vi "GetAppOutput.vi"(8 "error in (no error)":errorcluster, 11 "RingdownPlugin in":refnum<class "RingdownPlugin.lvclass">) -> (0 "error out":errorcluster, 3 "RingdownPlugin out":refnum<class "RingdownPlugin.lvclass">)   [LabVIEW 2014, in "AppPlugins.lvlib" / "RingdownPlugin.lvclass"]
uses:
  RingdownPlugin.lvclass
  TypeDef/RingdownOutput.ctl
  RingdownPlugin.lvclass/RingdownPlugin.ctl
  Accessors/Read RingdownConfig.vi
panel:
  out "Warning":i32
  out "Output Parameters":T1
  out "Time of process":dbl
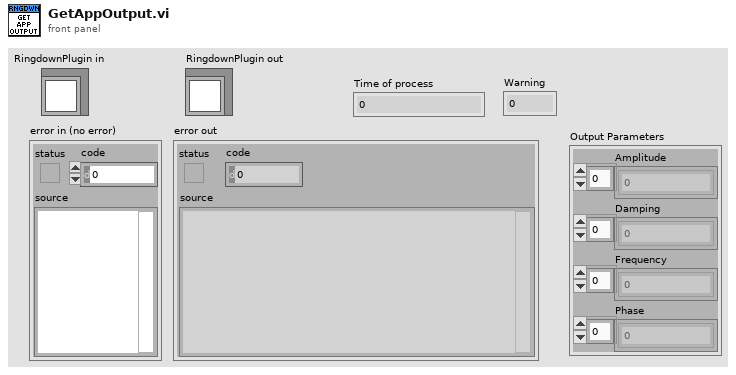
[diagram p1: front panel]
types:
  T1 = cluster{"Amplitude":dbl[], "Damping":dbl[], "Frequency":dbl[], "Phase":dbl[]}
  T2 = typedef "AppPlugins.lvlib/RingdownPlugin.lvclass/RingdownOutput.ctl" = cluster{"FramesPerSecond":dbl, "PronyEstimate":dbl[], "RingdownParameters":cluster{"Amplitude":dbl[], "Damping":dbl[], "Frequency":dbl[], "Phase":dbl[]}, "ReportingTime":dbl, "DataSize":u32, "InputSignal":dbl[]}
  T3 = typedef "AppPlugins.lvlib/RingdownPlugin.lvclass/RingdownConfig.ctl" = cluster{"Config":cluster{"Addmod":i32, "Scalmod":i32, "Lpocon":i32, "Pircon":i32, "Dmodes":i32, "Lpmcon":u16, "Lpacon":u16, "Fbcon":u16, "Ordcon":i32, "Trimre":dbl, "Ftrimh":dbl, "Ftriml":dbl}, "Window":cluster{"StOffset":i32, "EndOffset":i32, "Length":i32}, "V index":i32, "I index":i32, "PosSeq":bool}
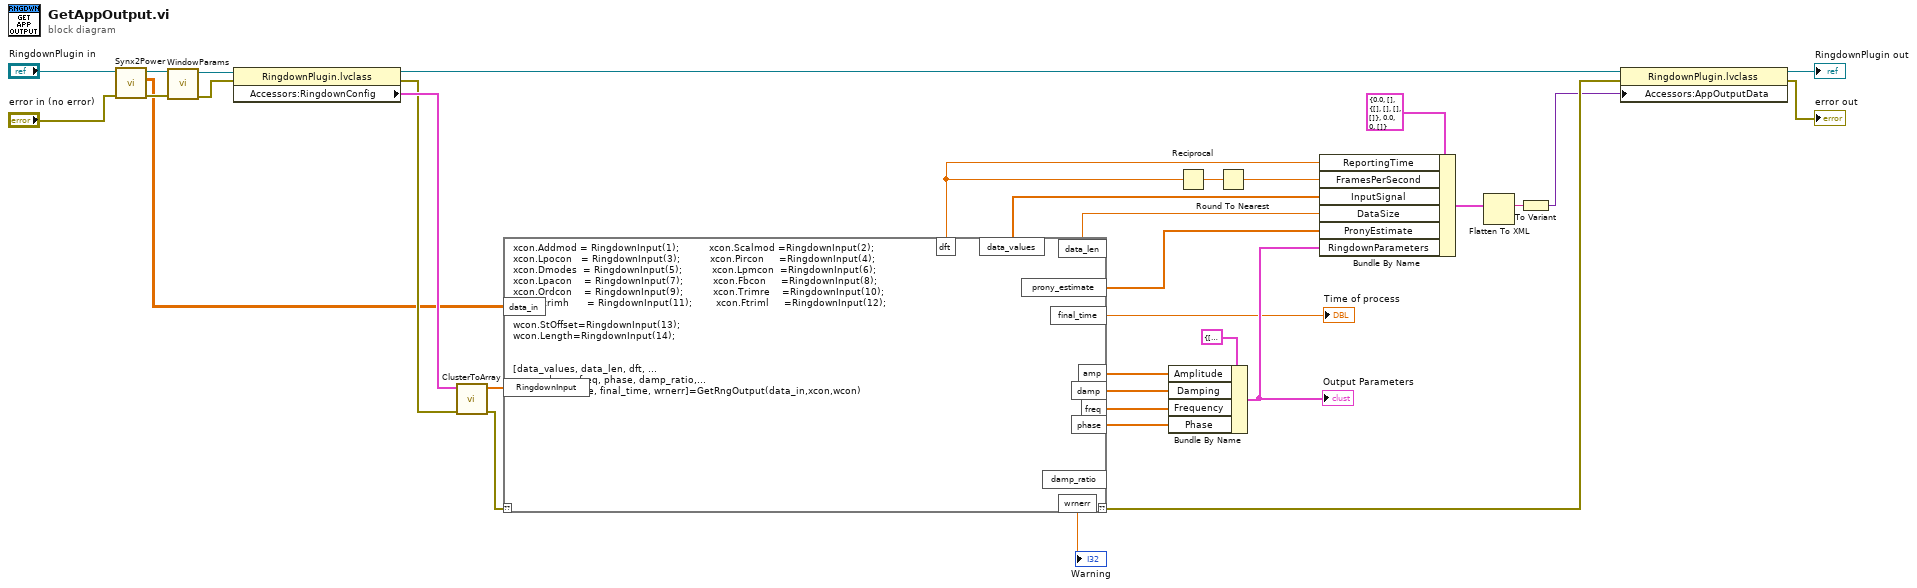
[diagram p0: block diagram]
diagram:
  n1 = call "Synx2Power.vi"("error in (no error)"="error in (no error)", "RingdownPlugin in"="RingdownPlugin in") -> ("error out"=w26:errorcluster, "Real Power"=w7:dbl[][], "RingdownPlugin out"=w25:refnum<class "RingdownPlugin.lvclass">)  [unwired: 6 in, 1 out]
  n2 = call "WindowParams.vi"("error in (no error)"=w26, "RingdownPlugin"=w25) -> ("error out"=w23:errorcluster, "RingdownPlugin.lvclass"=w24:refnum<class "RingdownPlugin.lvclass">)  [unwired: 8 in]
  n3 = property class="RingdownPlugin.lvclass"(reference=w24, error in=w23) -> (reference out=w22:refnum<class "RingdownPlugin.lvclass">, error out=w13:errorcluster, "Accessors:RingdownConfig"=w14:T3)
  n4 = call "ClusterToArray.vi"("error in (no error)"=w13, "RingdownConfig"=w14) -> ("error out"=w12:errorcluster, "RingdownInput"=w6:dbl[])  [unwired: 8 in]
  n5 = script code="xcon.Addmod = RingdownInput(1);          xcon.Scalmod =RingdownInput(2);        \nxcon.Lpocon   = RingdownInput(3);          xcon.Pircon     =RingdownInput(4);             \nxcon.Dmodes  = RingdownInput(5);          xcon.Lpmcon  =RingdownInput(6); \nxcon.Lpacon    = RingdownInput(7);          xcon.Fbcon     =RingdownInput(8);     \nxcon.Ordcon    = RingdownInput(9);          xcon.Trimre    =RingdownInput(10);          \nxcon.Ftrimh      = RingdownInput(11);        xcon.Ftriml     =RingdownInput(12); \n\nwcon.StOffset=RingdownInput(13);           \nwcon.Length=RingdownInput(14);  \n\n\n[data_values, data_len, dft, ...\n  amp, damp, freq, phase, damp_ratio,...\n  prony_estimate, final_time, wrnerr]=GetRngOutput(data_in,xcon,wcon)"("??"=w12, "data_in"=w7, "RingdownInput"=w6) -> ("??"=w4:errorcluster, "dft"=w19:dbl, "data_values"=w18:dbl[], "data_len"=w17:dbl, "prony_estimate"=w16:dbl[], "final_time"=→"Time of process":dbl, "amp"=w11:dbl[], "damp"=w10:dbl[], "freq"=w9:dbl[], "phase"=w8:dbl[], "wrnerr"=→"Warning":dbl)  [unwired: 1 out]
  n6 = Bundle By Name(cluster=T1 {"Amplitude"=[], "Damping"=[], "Frequency"=[], "Phase"=[0.0, 0.0, 0.0, 0.0, 0.0, 0.0, 0.0, 0.0, 0.0, 0.0, 0.0, 0.0, 0.0, 0.0, 0.0, 0.0]} ("RingdownParameters"), "Amplitude"=w11, "Damping"=w10, "Frequency"=w9, "Phase"=w8) -> (w21:T1)
  "Output Parameters" <- w21
  n7 = Reciprocal(x=w19) -> (1/x=w31:dbl)
  n8 = Round To Nearest(number=w31) -> (nearest integer value=w30:dbl)
  n9 = Bundle By Name(cluster=T2 {"FramesPerSecond"=0.0, "PronyEstimate"=[], "RingdownParameters"={"Amplitude"=[], "Damping"=[], "Frequency"=[], "Phase"=[]}, "ReportingTime"=0.0, "DataSize"=0, "InputSignal"=[]} ("RingdownOutput"), "ReportingTime"=w19, "FramesPerSecond"=w30, "InputSignal"=w18, "DataSize"=w17, "PronyEstimate"=w16, "RingdownParameters"=w21) -> (w3:T2)
  n10 = Flatten To XML(anything=w3) -> (xml string=w2:string)
  n11 = To Variant(anything=w2) -> (Variant=w1:variant)
  n12 = property class="RingdownPlugin.lvclass"(reference=w22, error in=w4, "Accessors:AppOutputData"=w1) -> (reference out=→"RingdownPlugin out":refnum<class "RingdownPlugin.lvclass">, error out=→"error out":errorcluster)
